vi "SQL写入.vi"(0 "WorkNumber":string, 1 "ProductNumber":string, 3 "TestMessage":string, 4 "ProssureType":string, 5 "error in (no error)":errorcluster caption="错误输入（无错误）", 6 "ADODB._Connection In":refnum<k7>, 7 "Workorder":string) -> (14 "ADODB._Connection Out":refnum<k7>, 19 "error out":errorcluster caption="错误输出")   [LabVIEW 2017]
panel:
  out "连接的字符串":string
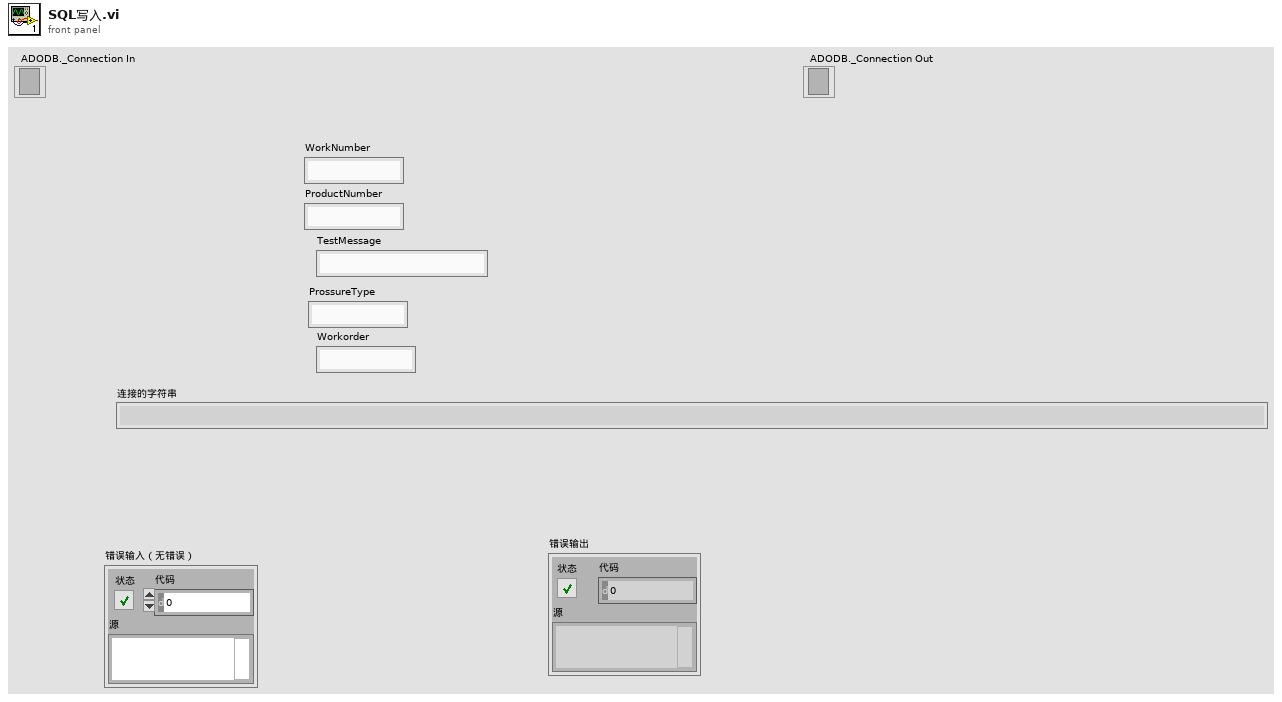
[diagram p1: front panel]
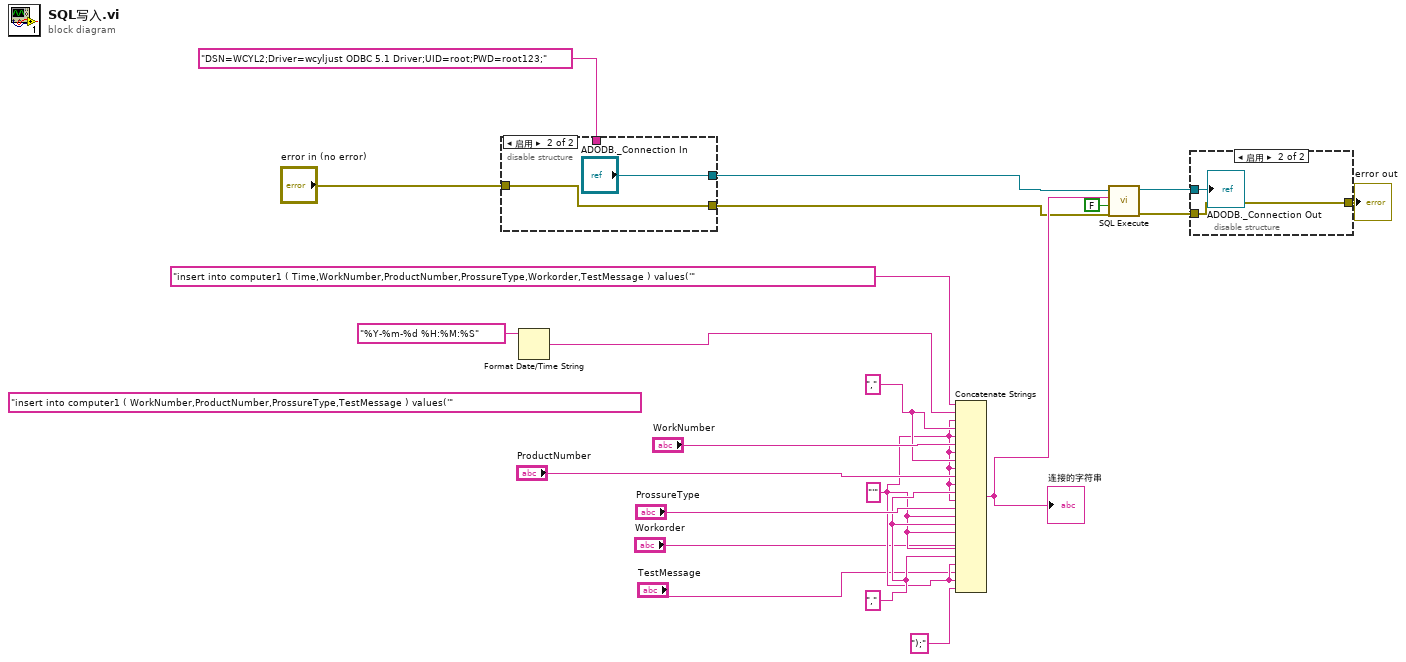
[diagram p0: block diagram]
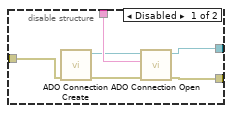
[diagram p2: hidden frame]
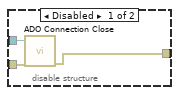
[diagram p3: hidden frame]
diagram:
  (unwired) "insert into computer1 ( WorkNumber,ProductNumber,ProssureType,TestMessage ) values('" ("Command Text")
  w3 = "'" ("字符串")
  w9 = "," ("字符串")
  w11 = "," ("字符串")
  n1 = disable-structure shown="启用" {
    disable-tunnel: "DSN=WCYL2;Driver=wcyljust ODBC 5.1 Driver;UID=root;PWD=root123;" ("ConnectionString") -> [w27 _]
    disable-tunnel: "error in (no error)" -> [w26 w28]
    disable-tunnel: [w23 "ADODB._Connection In"] -> w5
    disable-tunnel: [w22 w28] -> w4
    frame Disabled {
      n2 = call <userlib>:"ADO Connection Create.vi"("error in (no error)"=w26) -> ("error out"=w24:errorcluster, "ADODB._Connection Out"=w25:refnum<k7>)  [unwired: 9 in]
      n3 = call <userlib>:"ADO Connection Open.vi"("error in (no error)"=w24, "ConnectionString"=w27, "ADODB._Connection In"=w25) -> ("error out"=w22:errorcluster, "ADODB._Connection Out"=w23:refnum<k7>)  [unwired: 7 in]
    }
    frame Enabled {
    }
  }
  n4 = Format Date/Time String(time format string (%c)="%Y-%m-%d %H:%M:%S" ("时间格式字符串(%c)")) -> (date/time string=w12:string)  [unwired: 2 in]
  n5 = Concatenate Strings("insert into computer1 ( Time,WorkNumber,ProductNumber,ProssureType,Workorder,TestMessage ) values('" ("Command Text"), w12, w3, w11, w3, "WorkNumber", w3, w11, w3, "ProductNumber", w3, w9, w3, "ProssureType", w3, w9, w3, "Workorder", w3, w9, w3, "TestMessage", w3, ");" ("字符串")) -> (w17:string)
  "连接的字符串" <- w17
  n6 = call <userlib>:"SQL Execute.vi"("error in (no error)"=w4, "Return Data (T)"=FALSE, "Command Text"=w17, "ADODB._Connection In"=w5) -> ("error out"=w7:errorcluster, "ADODB._Connection Out"=w8:refnum<k7>)  [unwired: 4 in, 2 out]
  n7 = disable-structure shown="启用" {
    disable-tunnel: [w32 w34] -> w15
    disable-tunnel: w8 -> [w31 w33]
    disable-tunnel: w7 -> [w30 w34]
    frame Disabled {
      n8 = call <userlib>:"ADO Connection Close.vi"("error in (no error)"=w30, "ADODB._Connection In"=w31) -> ("error out"=w32:errorcluster)  [unwired: 8 in, 1 out]
    }
    frame Enabled {
      "ADODB._Connection Out" <- w33
    }
  }
  "error out" <- w15
